vi "Dashboard Main.vi"() -> ()   [LabVIEW 2011]
uses:
  <vilib>/Rock Robotics/WPI/Camera/WPI_CameraImageSize.ctl
  Dashboard Datatype.ctl
  <vilib>/Rock Robotics/WPI/DriverStation/WPI_DriverStationDigitalData.ctl
  UDP Communication Folder/UDP Dashboard Packet TypeDef.ctl
panel:
  out "Turret Pot":dbl(knob) scale=0.0..5.0
  out "Right":bool
  out "Off":bool
  out "Left":bool
  in  "Tab Control":enum32{"Competition", "Debug"}(tab)
  out "Aligned":bool
  in  "RPM":dbl(slide)=-30.0 scale=-200.0..200.0 scale format="%#.2g"
  out "Warmup":bool
  out "Automatic Mode":bool
  out "Allow Fire":bool
  in  "Viewer":T1(tab)
  in  "Video Enable":bool=TRUE
  out "Camera Image":T2(plugin-control)
  out "Buttons 1":cluster{"1":bool, "2":bool, "3":bool}
  out "Kinect 1":cluster{"X":dbl, "Y":dbl, "Z":dbl} {"X" scale=1.0..-1.0; "Y" scale=1.0..-1.0; "Z" scale=1.0..-1.0}
  out "Buttons 2":cluster{"1":bool, "2":bool, "3":bool}
  out "Kinect 2":cluster{"X":dbl, "Y":dbl, "Z":dbl} {"X" scale=1.0..-1.0; "Y" scale=1.0..-1.0; "Z" scale=1.0..-1.0}
  out "Version":string
  out "Skeleton Picture":picture
  out "Players":i8
  out "Processed Image":T2(plugin-control)
  in  "Display Mask":bool
  in  "Particle Count Limit":i32=10
  in  "Image Size":T3=enum."320x240"
  out "Distance":dbl format="%.2g"
  out "Gear":i32 format="%#.0f"
  out "Camera Tracking":bool
  out "Gyro":dbl(knob) scale=0.0..360.0
  out "Gyro Angle":dbl
  out "# Balls":u32
  in  "?":T4(tab)
  out "Encoders":cluster{"Average":dbl, "Left":dbl, "Right":dbl}
  out "IR Values":T5
  out "UDP Reading":bool
  out "Turret Info":T6 {"Target Pot" scale=1.0..4.0; "Current Voltage" scale=1.0..4.0}
  out "Gyro Angle":dbl(knob) scale=0.0..360.0
  out "Shooter Info":T7
  out "Solenoids":T8
  out "Ball State Machine":T9
  in  "Display Mask":bool
  in  "Color Range":T10={"Hue"={"Lower"=120, "Upper"=137}, "Sat"={"Lower"=130, "Upper"=255}, " Luma"={"Lower"=100, "Upper"=255}}
  in  "Score Limits":T11={"Rect Coverage"=66.0, "Aspect Ratio"=70.0, "X Edge Strength"=40.0, "Y Edge Strength"=60.0}
  out "Camera Image 2":T2(plugin-control)
  out "Processed Image 2":T2(plugin-control)
  out "Tracking Setpoint":dbl
  in  "Tracking Constant":dbl=0.07
  in  "Tracking Tolerance":dbl=0.2
  in  "Color":u32(colorbox)=16711680
  in  "Left Offset Percentage":dbl=2.4
  out "Gyro Angle 2":dbl
  out "Tracking OUT":dbl
  out "Target Info":T12(array[cluster])
  out "Servo Positions In":cluster{"X":dbl, "Y":dbl}
  in  "Area Size Limit":i32=444
  in  "Decimation":i32=1
  in  "Shooter PID gains":T13={"proportional gain (Kc)"=0.0025, "integral time (Ti, min)"=0.007, "derivative time (Td, min)"=0.0}
  in  "Tracking PID gains":T13={"proportional gain (Kc)"=0.25, "integral time (Ti, min)"=0.01, "derivative time (Td, min)"=0.0015}
  in  "Shooter PID gains 2":T13={"proportional gain (Kc)"=0.0028, "integral time (Ti, min)"=0.0, "derivative time (Td, min)"=0.0}
  in  "Shooter Control":T14={"Manual Enabled"=FALSE, "Manual Distance"=0.0, "Power Constant"=0.0, "RPM Constant"=-30.0, "Layup Distance"=10.0, "RPM Range"={"Max Percentage"=1.005, "Min Percentage"=0.985}, "Dt In"=0.02}
  in  "Tracking Limit":dbl=0.55
  in  "Autonomous Ball Collection / Shoot Period":dbl=7.0
  out "8 -- Battery":sgl(graph)
  out "Analog Input":sgl[](array[slide]) scale=0.0..5.0
  out "Dashboard Datatype Warning":string="Warning: The Dashboard Datatype used by the robot project and this dashboard do not match.\nSee diagram for more details."
  out "Robot IP Address":string
  out "Image Error Message":string="Timeout in Camera Communications"
  out "Solenoid Output":bool[](array[boolean])
  out "PWM":cluster{u8, u8}[](array[slide])=[{0, 157}, {0, 157}, {0, 157}, {0, 157}, {0, 157}, {0, 157}, {0, 157}, {0, 157}, {0, 157}, {0, 169}] scale=1.0..255.0
  out "GPIO Output Enable":bool[](array[boolean])
  out "GPIO State":bool[](array[boolean])
  out "Relay":cluster{"Forward":bool[], "Reverse":bool[]}
  # "Layup"
  # "FAST - LONG"
  # "SLOW - SHORT"
  # "Gyro"
  # "SHOOTING PID"
  # "WARM UP PID"
  # "PID Values:\n   2.28.12:  0.003, 0, 0\n   3.2.12:    0.006, 0.000001, 0.0001\n   3.11.12:  0.0025, 0.009, 0\n   3.12.12: 0.0025, 0.007, 0"
  # "PID Values:\n   3.12.12: 2.5, 0.009, 0  Oscillating\n   3.12.12: 4.0, 0, 0         Steady state error\n\n   3.30.12: 0.03, 0.01, 0.002 (gyro)\n   4.26.12: 0.27, 0.01, 0.0018 (okay..)"
  # "PID Values:\n   3.12.12: 0.0028, 0, 0"
  # "Seconds"
  # "Limits tracking pid output"
  # "Analog #1"
  # "1"
  # "7"
  # "Communications"
  # "Solenoid #1"
  # "1"
  # "8"
  # "Digital #1"
  # "1"
  # "10"
  # "1"
  # "14"
  # "1"
  # "8"
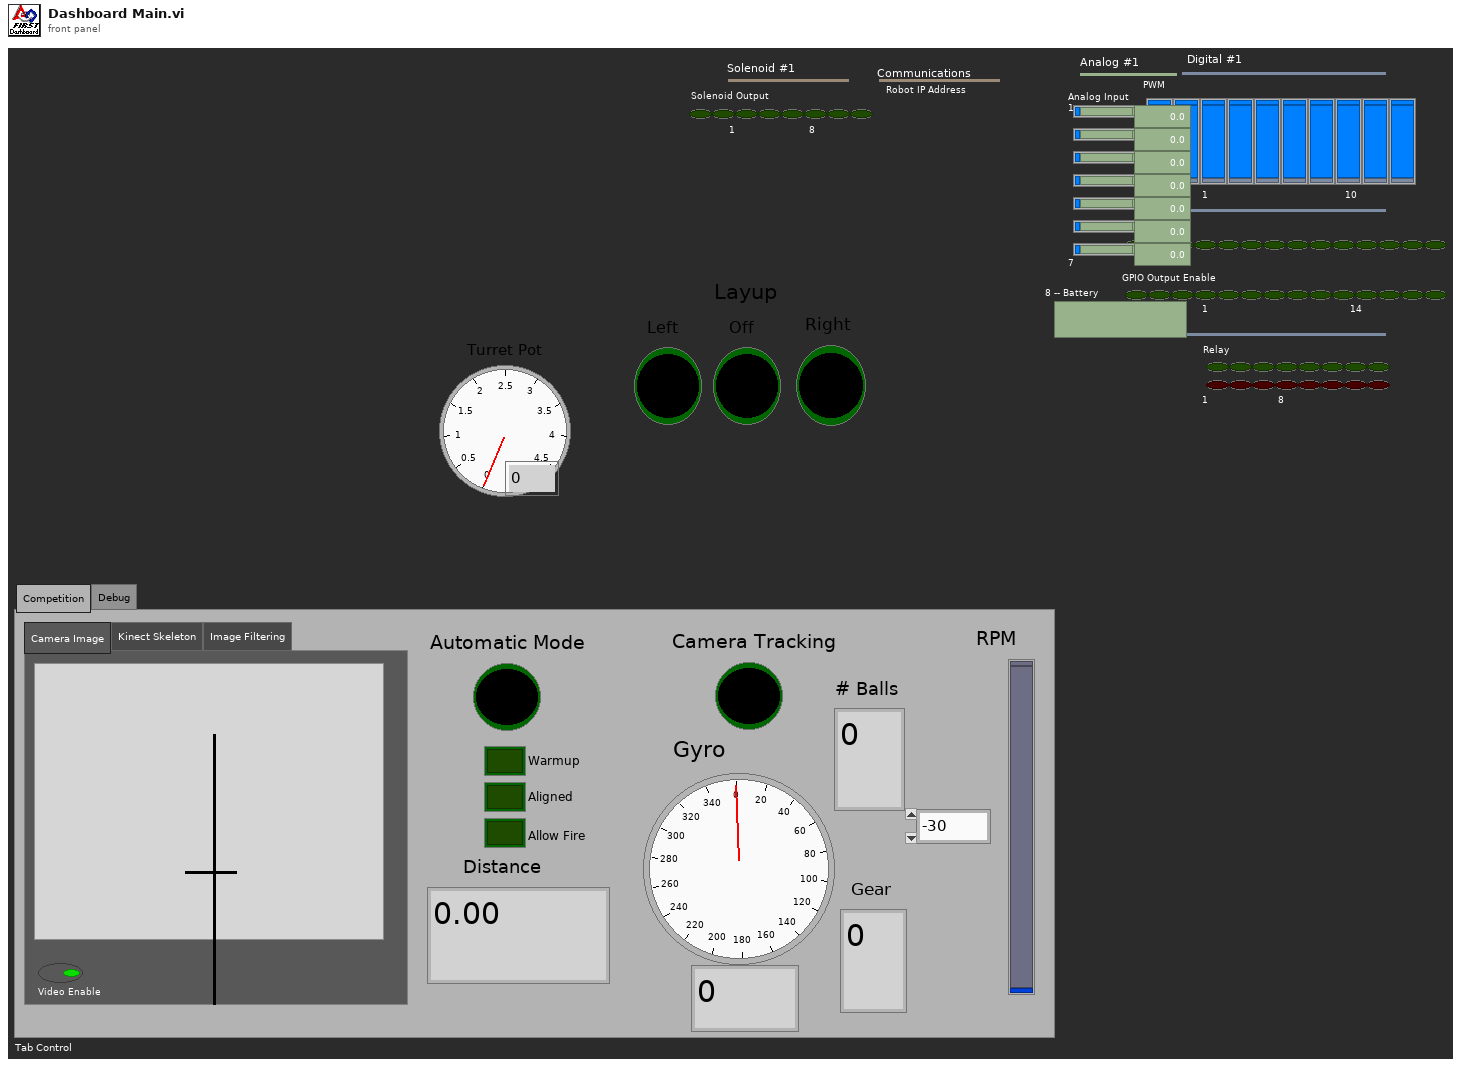
[diagram p1: front panel]
types:
  T1 = enum32{"Camera Image", "Kinect Skeleton", "Image Filtering"}
  T2 = typedef "IMAQ Image.ctl" = refnum<image>
  T3 = typedef "WPI_CameraImageSize.ctl" = enum16{"640x480", "320x240", "160x120"}
  T4 = enum32{"Sensors", "Vision Calib", "Vision Readings", "Numeric Controls"}
  T5 = cluster{"Front Roller":bool, "Back Roller":bool, "Lower Mag":bool, "Upper Mag":bool, "Front Enter":bool, "Rear Enter":bool}
  T6 = cluster{"Target Pot":dbl, "Motor Output":dbl, "Current Voltage":dbl}
  T7 = cluster{"Current RPM":dbl, "Distance Setpoint":dbl, "Target RPM":dbl, "Motor Output":dbl, "Base Power":dbl, "Dt Out":dbl}
  T8 = cluster{"Gear Shifter":bool, "Tipper":bool, "Tipper Lock":bool, "Stabilizer":bool}
  T9 = cluster{"Current State":u32, "Reading State":u32, "Number of Balls":u32, "State":enum16{"Load Balls", "Shoot", "Wait"}}
  T10 = cluster{"Hue":cluster{"Lower":i32, "Upper":i32}, "Sat":cluster{"Lower":i32, "Upper":i32}, " Luma":cluster{"Lower":i32, "Upper":i32}}
  T11 = cluster{"Rect Coverage":dbl, "Aspect Ratio":dbl, "X Edge Strength":dbl, "Y Edge Strength":dbl}
  T12 = cluster{"Position":cluster{"X":dbl, "Y":dbl}, "Distance (ft)":dbl}[]
  T13 = cluster{"proportional gain (Kc)":dbl, "integral time (Ti, min)":dbl, "derivative time (Td, min)":dbl}
  T14 = cluster{"Manual Enabled":bool, "Manual Distance":dbl, "Power Constant":dbl, "RPM Constant":dbl, "Layup Distance":dbl, "RPM Range":cluster{"Max Percentage":dbl, "Min Percentage":dbl}, "Dt In":dbl}
  T15 = typedef "UDP Dashboard Packet TypeDef.ctl" = cluster{"Distance":dbl, "Shooter Control":cluster{"Manual Enabled":bool, "Manual Distance":dbl, "Power Constant":dbl, "RPM Constant":dbl, "Layup Distance":dbl, "RPM Range":cluster{"Max Percentage":dbl, "Min Percentage":dbl}, "Dt In":dbl}, "Tracking Setpoint":dbl, "Shooter PID gains":cluster{"proportional gain (Kc)":dbl, "integral time (Ti, min)":dbl, "derivative time (Td, min)":dbl}, "Tracking PID gains":cluster{"proportional gain (Kc)":dbl, "integral time (Ti, min)":dbl, "derivative time (Td, min)":dbl}, "Shooter PID gains 2":cluster{"proportional gain (Kc)":dbl, "integral time (Ti, min)":dbl, "derivative time (Td, min)":dbl}, "Tracking Tolerance":dbl, "Tracking Limit":dbl, "Autonomous Ball Collection / Shoot Period":dbl}
  T16 = typedef "Dashboard Datatype.ctl" = cluster{cluster{"AnalogModule[0]":cluster{"Channel[0]":sgl, "Channel[1]":sgl, "Channel[2]":sgl, "Channel[3]":sgl, "Channel[4]":sgl, "Channel[5]":sgl, "Channel[6]":sgl, "Channel[7]":sgl}, "AnalogModule[1]":cluster{"Channel[0]":sgl, "Channel[1]":sgl, "Channel[2]":sgl, "Channel[3]":sgl, "Channel[4]":sgl, "Channel[5]":sgl, "Channel[6]":sgl, "Channel[7]":sgl}}, cluster{"DigitalModule[0]":T17, "DigitalModule[1]":T17}, "Solenoid":u8, "IR Values":cluster{"Front Roller":bool, "Back Roller":bool, "Lower Mag":bool, "Upper Mag":bool, "Front Enter":bool, "Rear Enter":bool}, "Solenoids":cluster{"Gear Shifter":bool, "Tipper":bool, "Tipper Lock":bool, "Stabilizer":bool}, "Allow Fire":bool, "Encoders":cluster{"Average":dbl, "Left":dbl, "Right":dbl}, "UDP Reading":bool, "Turret Info":cluster{"Target Pot":dbl, "Motor Output":dbl, "Current Voltage":dbl}, "Shooter Controls":cluster{"Shooter Warmup":bool, "Shooter Allow Fire":bool}, "Automatic Mode":bool, "Gyro Angle":dbl, "Servo Positions In":cluster{"X":dbl, "Y":dbl}, "Layup State":enum16{"Layup Left", "Layup Right", "Off"}, "Shooter Info":cluster{"Current RPM":dbl, "Distance Setpoint":dbl, "Target RPM":dbl, "Motor Output":dbl, "Base Power":dbl, "Dt Out":dbl}, "Tracking":bool, "Ball State Machine":cluster{"Current State":u32, "Reading State":u32, "Number of Balls":u32, "State":enum16{"Load Balls", "Shoot", "Wait"}}}
  T17 = typedef "WPI_DriverStationDigitalData.ctl" = cluster{"Relay Fwd":u8, "Relay Rev":u8, "GPIO":u16, "GPIO_OE":u16, "PWM":cluster{"PWM[0]":u8, "PWM[1]":u8, "PWM[2]":u8, "PWM[3]":u8, "PWM[4]":u8, "PWM[5]":u8, "PWM[6]":u8, "PWM[7]":u8, "PWM[8]":u8, "PWM[9]":u8}}
  T18 = typedef "Image Type" = u32
  T19 = cluster{"Competition mode":bool, "Robot Link":bool, "Autonomous":bool, "Enabled":bool, "E-Stop":bool}
  T20 = cluster{"AnalogModule[0]":cluster{"Channel[0]":sgl, "Channel[1]":sgl, "Channel[2]":sgl, "Channel[3]":sgl, "Channel[4]":sgl, "Channel[5]":sgl, "Channel[6]":sgl, "Channel[7]":sgl}, "AnalogModule[1]":cluster{"Channel[0]":sgl, "Channel[1]":sgl, "Channel[2]":sgl, "Channel[3]":sgl, "Channel[4]":sgl, "Channel[5]":sgl, "Channel[6]":sgl, "Channel[7]":sgl}}
  T21 = cluster{"DigitalModule[0]":T17, "DigitalModule[1]":T17}
  T22 = cluster{"Shooter Warmup":bool, "Shooter Allow Fire":bool}
  T23 = cluster{"Channel[0]":sgl, "Channel[1]":sgl, "Channel[2]":sgl, "Channel[3]":sgl, "Channel[4]":sgl, "Channel[5]":sgl, "Channel[6]":sgl, "Channel[7]":sgl}[]
  T24 = cluster{"Channel[0]":sgl, "Channel[1]":sgl, "Channel[2]":sgl, "Channel[3]":sgl, "Channel[4]":sgl, "Channel[5]":sgl, "Channel[6]":sgl, "Channel[7]":sgl}
  T25 = typedef "LVRectTypeDef.ctl" = cluster{"left":i16, "top":i16, "right":i16, "bottom":i16}
  T26 = typedef "SkeletonTrackState.ctl" = enum32{"NotTracked", "PositionOnly", "Tracked"}
  T27 = cluster{"TrackingState":u8[], "Position":cluster{"x":sgl, "y":sgl, "z":sgl}, cluster{"x":sgl, "y":sgl, "z":sgl, sgl}[], "TrackState":T26}
  T28 = cluster{cluster{"ScaledToPercentRange":dbl, "ScaledToPercentRange":dbl, "ScaledToPercentRange":dbl}, cluster{bool, bool, bool}}[]
  T29 = typedef "LVBoundsTypeDef.ctl" = cluster{"Width":u32, "Height":u32}
  T30 = cluster{cluster{"ScaledToPercentRange":dbl, "ScaledToPercentRange":dbl, "ScaledToPercentRange":dbl}, cluster{bool, bool, bool}}
  T31 = cluster{"ScaledToPercentRange":dbl, "ScaledToPercentRange":dbl, "ScaledToPercentRange":dbl}
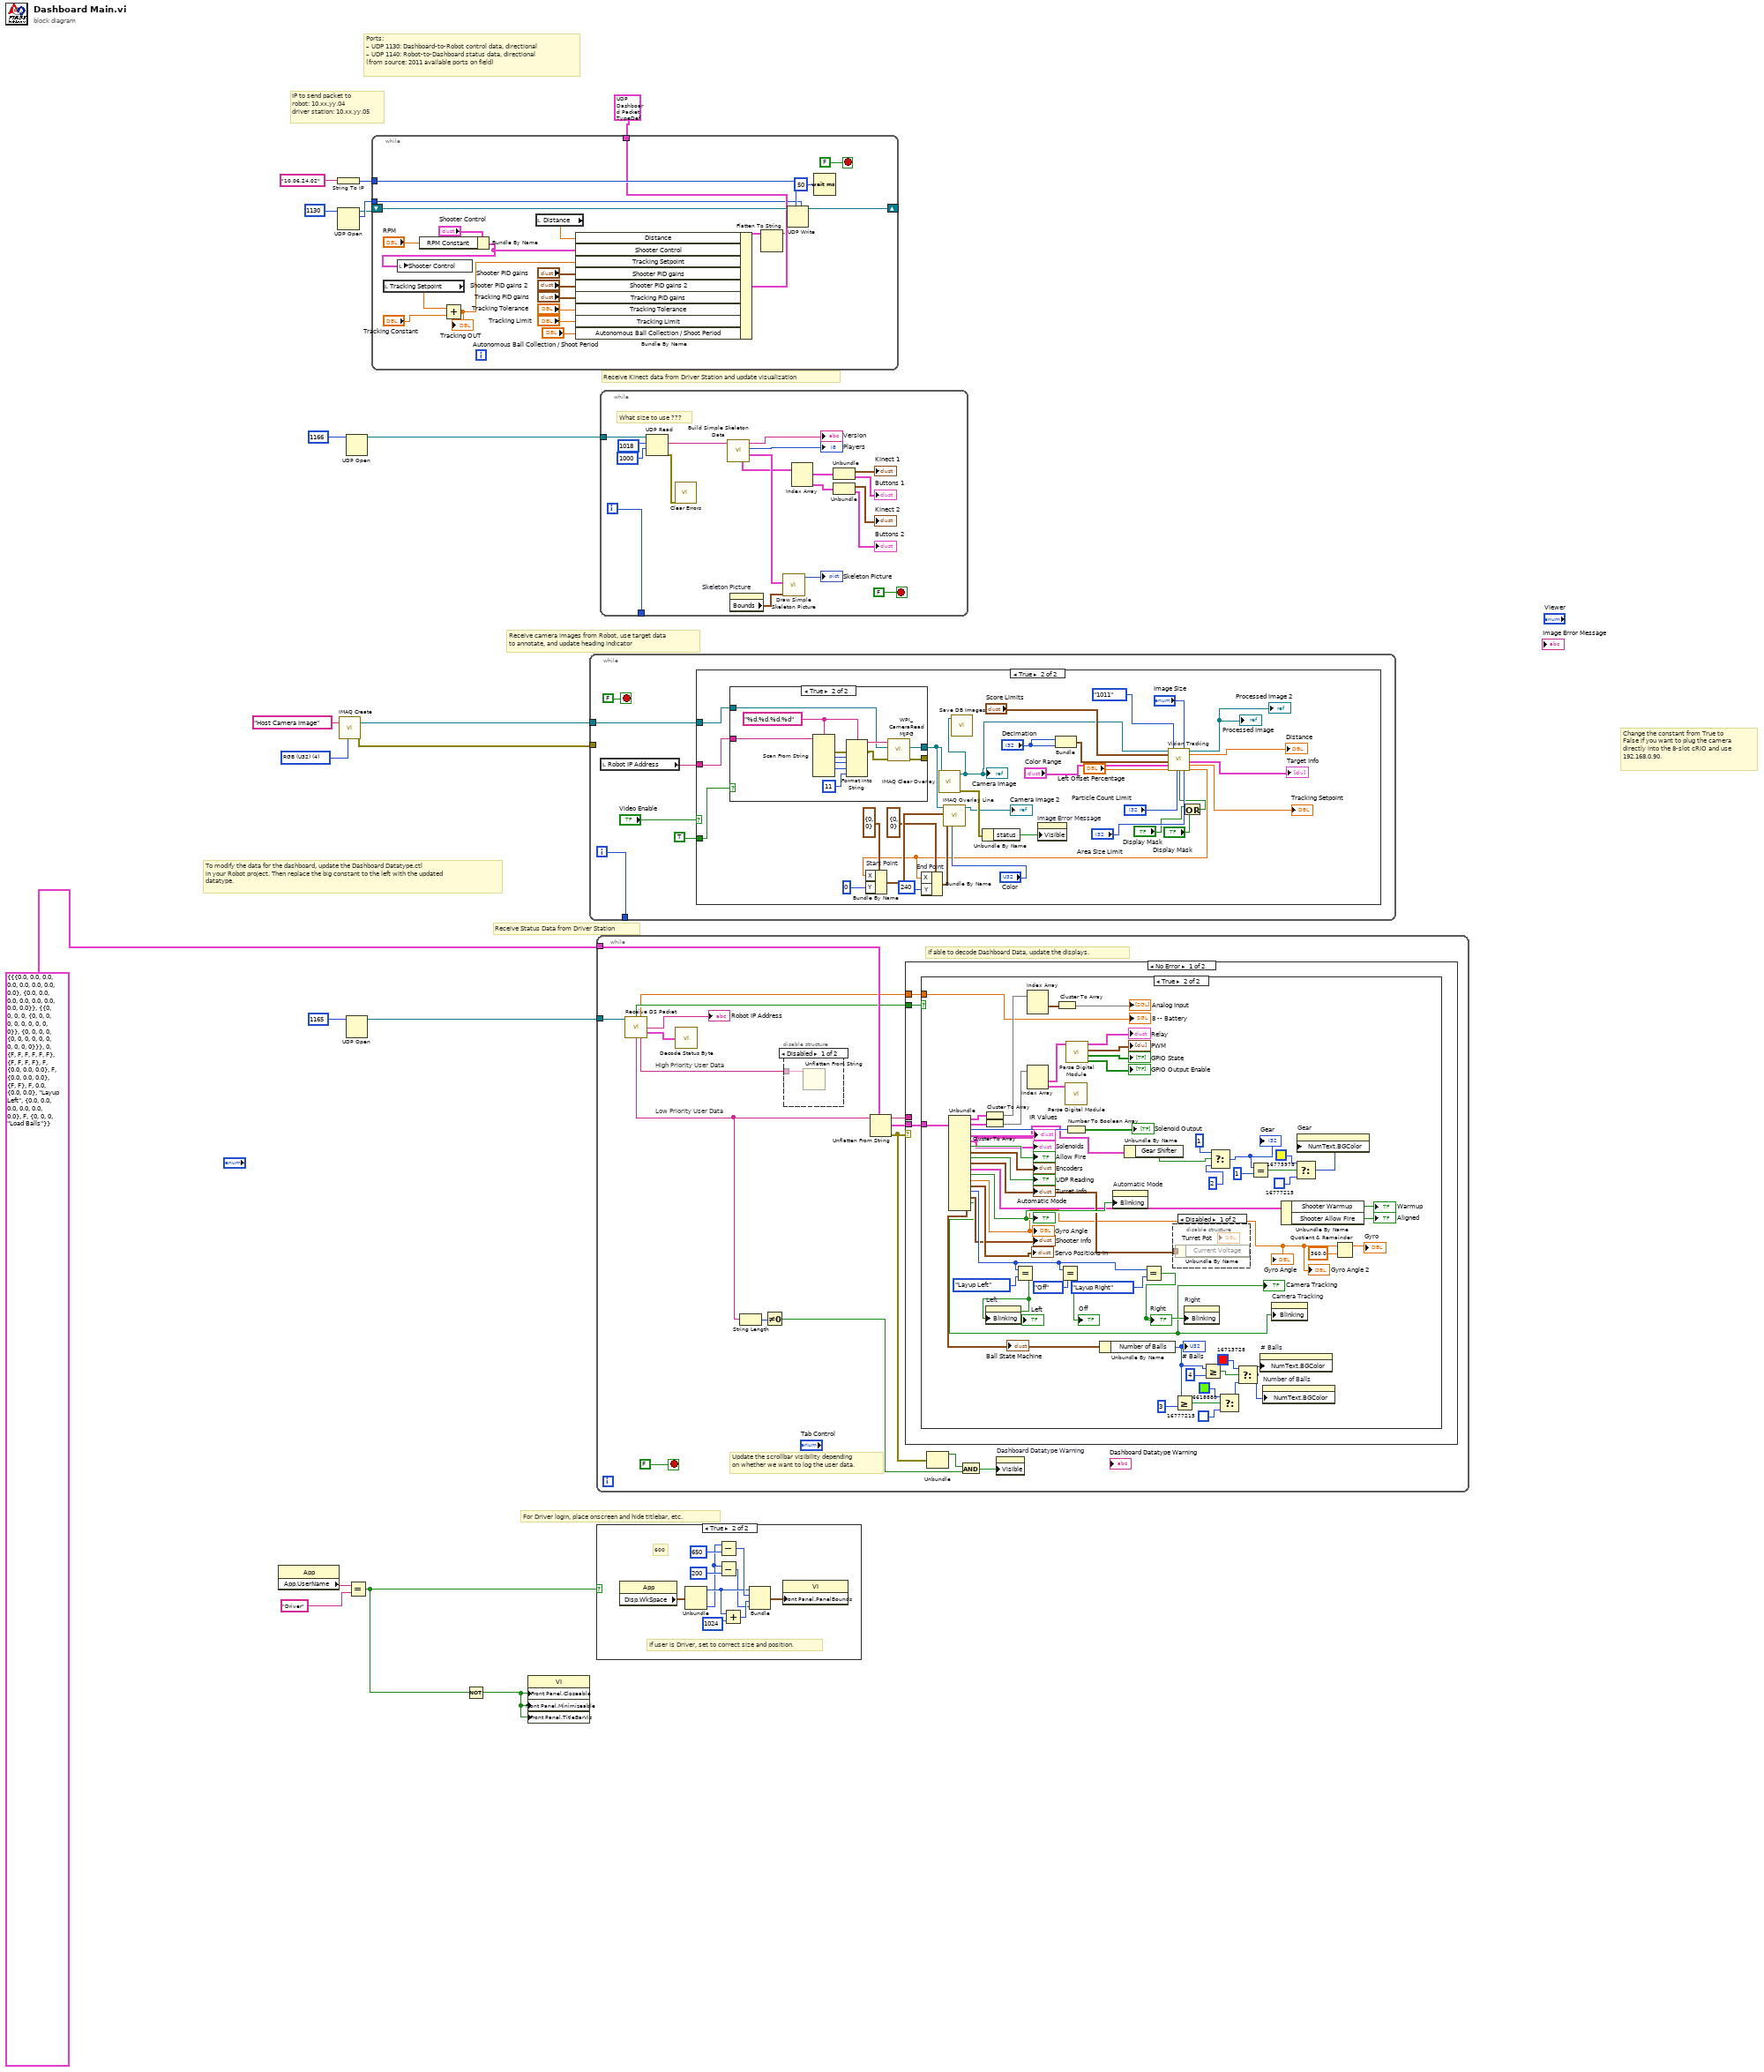
[diagram p0: block diagram]
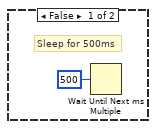
[diagram p7: hidden frame]
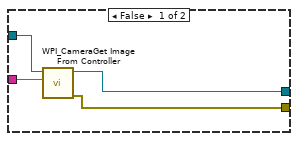
[diagram p8: hidden frame]
diagram:
  w17 = T18 4 items=["Grayscale (U8)", "Grayscale (I16)", "Grayscale (SGL)", "Complex (CSG)", "RGB (U32)", "HSL (U32)", "RGB (U64)"] ("Image Type")
  # "IP to send packet to \nrobot: 10.xx.yy.04\ndriver station: 10.xx.yy.05"
  # "Ports:\n– UDP 1130: Dashboard-to-Robot control data, directional\n– UDP 1140: Robot-to-Dashboard status data, directional\n(from source: 2011 available ports on field)"
  # "Change the constant from True to\nFalse if you want to plug the camera\ndirectly into the 8-slot cRIO and use\n192.168.0.90."
  # "Receive Kinect data from Driver Station and update visualization"
  # "For Driver login, place onscreen and hide titlebar, etc."
  # "To modify the data for the dashboard, update the Dashboard Datatype.ctl\nin your Robot project. Then replace the big constant to the left with the updated\ndatatype."
  # "Receive Status Data from Driver Station"
  # "Receive camera images from Robot, use target data\nto annotate, and update heading indicator"
  n1 = property class="App"() -> ("App.UserName"=w12:string)  [unwired: 2 in, 2 out]
  n2 = String To IP(1:"10.06.24.02") -> (0:w1:u32)
  n3 = UDP Open(11:u16 1130 ("port")) -> (port=w2:refnum<k16>, 2:w3:u16)  [unwired: 2 in, 3 out]
  n4 = call "IMAQ Create"("Image Name"="Host Camera Image", "Image Type"=w17) -> ("New Image"=w15:T2, "error out"=w14:errorcluster)  [unwired: 2 in, 1 out]
  n5 = UDP Open(11:u16 1166 ("port")) -> (port=w8:refnum<k16>)  [unwired: 2 in, 4 out]
  n6 = UDP Open(11:u16 1165 ("port")) -> (port=w18:refnum<k16>)  [unwired: 2 in, 4 out]
  n7 = Equal?(x=w12, y="Driver") -> (x = y?=w11:bool)
  n8 = while {
    tunnel: w1 -> [w39]
    tunnel: T15 {"Distance"=0.0, "Shooter Control"={"Manual Enabled"=FALSE, "Manual Distance"=0.0, "Power Constant"=0.0, "RPM Constant"=0.0, "Layup Distance"=0.0, "RPM Range"={"Max Percentage"=0.0, "Min Percentage"=0.0}, "Dt In"=0.0}, "Tracking Setpoint"=0.0, "Shooter PID gains"={"proportional gain (Kc)"=0.0, "integral time (Ti, min)"=0.0, "derivative time (Td, min)"=0.0}, "Tracking PID gains"={"proportional gain (Kc)"=0.0, "integral time (Ti, min)"=0.0, "derivative time (Td, min)"=0.0}, "Shooter PID gains 2"={"proportional gain (Kc)"=0.0, "integral time (Ti, min)"=0.0, "derivative time (Td, min)"=0.0}, "Tracking Tolerance"=0.0, "Tracking Limit"=0.0, "Autonomous Ball Collection / Shoot Period"=0.0} ("UDP Dashboard Packet") -> [w38]
    tunnel: w3 -> [w35]
    shift-right: [w34] -> _
    shift-left: w2 -> [w40]
    stop <- FALSE stop-if-true
    n9 = local read "Tracking Setpoint"() -> (w24:dbl)
    n10 = Bundle By Name(cluster="Shooter Control", "RPM Constant"="RPM") -> (w26:T14)
    n11 = local write "Shooter Control"(w26) -> ()
    n12 = Add(x=w24, y="Tracking Constant") -> (x+y=w23:dbl)
    "Tracking OUT" <- w23
    n13 = local read "Distance"() -> (w32:dbl)
    n14 = Bundle By Name(cluster=w38, "Distance"=w32, "Shooter Control"=w26, "Tracking Setpoint"=w23, "Shooter PID gains"="Shooter PID gains", "Shooter PID gains 2"="Shooter PID gains 2", "Tracking PID gains"="Tracking PID gains", "Tracking Tolerance"="Tracking Tolerance", "Tracking Limit"="Tracking Limit", "Autonomous Ball Collection / Shoot Period"="Autonomous Ball Collection / Shoot Period") -> (w37:T15)
    n15 = Flatten To String(anything=w37) -> (data string=w36:string)  [unwired: 3 in, 2 out]
    n16 = UDP Write(address=w39, port or service name=w35, connection ID=w40, data in=w36) -> (3:w34:refnum<k16>)  [unwired: 2 in, 1 out]
    n17 = Wait (ms)(milliseconds to wait=u32 50) -> ()  [unwired: 1 out]
  }
  n18 = Not(x=w11) -> (.not. x?=w10:bool)
  n19 = property class="VI"("Front Panel.Closeable"=w10, "Front Panel.Minimizeable"=w10, "Front Panel.TitleBarVis"=w10) -> ()  [unwired: 2 in, 2 out]
  n20 = while {
    tunnel: w15 -> [w45]
    tunnel: w14 -> [_]
    tunnel: [w42] -> _
    i -> [w42]
    stop <- FALSE stop-if-true
    n21 = local read "Robot IP Address"() -> (w46:string)
    n22 = case shown="True" "Video Enable" {
      tunnel: w46 -> [_ w80]
      tunnel: w45 -> [_ w79]
      tunnel: TRUE -> [_ w76]
      frame False {
        # "Sleep for 500ms"
        n23 = Wait Until Next ms Multiple(millisecond multiple=u32 500) -> ()  [unwired: 1 out]
      }
      frame True {
        n24 = case shown="True" w76 {
          tunnel: w79 -> [w83 w90]
          tunnel: [w81 w88] -> _
          tunnel: [w82 w89] -> w60
          tunnel: w80 -> [w84 w93]
          frame False {
            n25 = call <vilib>:"WPI_CameraGet Image From Controller.vi"("Controller Address"=w84, "Image"=w83) -> ("error out"=w81:errorcluster, "Image Out"=w82:T2)  [unwired: 2 in, 6 out]
          }
          frame True {
            w85 = "%d.%d.%d.%d" ("format string")
            n26 = Scan From String(format string=w85, input string=w93) -> (error out=w92:errorcluster, output 1=w94:i32, output 2=w95:i32, output 3=w96:i32)  [unwired: 2 in, 7 out]
            n27 = Format Into String(format string=w85, error in=w92, w94, w95, w96, 11 ("IP Suffix:")) -> (resulting string=w91:string, error out=w87:errorcluster)  [unwired: 1 in]
            n28 = call <vilib>:"WPI_CameraRead MJPG.vi"("error in"=w87, "Image"=w90, "address"=w91) -> ("error out"=w88:errorcluster, "Image Out"=w89:T2)  [unwired: 7 in]
          }
        }
        n29 = call "IMAQ Clear Overlay"("Image"=w60) -> ("error out"=w77:errorcluster, "Image Out"=w59:T2)  [unwired: 2 in, 7 out]
        "Camera Image" <- w59
        n30 = call "Save DB Images.vi"("Image"=w59) -> ()  [unwired: 2 in, 1 out]
        n31 = Unbundle By Name(w77) -> ("status"=w78:bool)
        n32 = property on="Image Error Message" class="Str"("Visible"=w78) -> ()  [unwired: 2 in, 2 out]
        n33 = Bundle("Decimation"="Decimation", "Decimation"="Decimation") -> (w69:cluster{"Decimation":i32, "Decimation":i32})  [unwired: 1 in]
        n34 = Or(x="Display Mask", y="Display Mask") -> (x .or. y?=w62:bool)
        n35 = call "Vision Tracking.vi"("Color Image In"=w59, "Score Limits"="Score Limits", "Decimate by"=w69, "Color Range"="Color Range", "Left Offset Percentage"="Left Offset Percentage", "Camera Type"=enum16{"206", "1011"}."1011", "Particle Count Limit"="Particle Count Limit", "Display Mask"=w62, "Image Size"="Image Size", "Area Size Limit"="Area Size Limit") -> ("Processed Image"=→"Processed Image" →"Processed Image 2":T2, "Distance (ft)"=→"Distance":dbl, "Target Info"=→"Target Info":T12, "Position.X"=→"Tracking Setpoint":dbl, "Center Line X"=w50:dbl)  [unwired: 5 in]
        n36 = Bundle By Name "Start Point"(cluster=cluster{"X":i32, "Y":i32} {"X"=0, "Y"=0} ("Start Point"), "X"=w50, "Y"=0) -> (w56:cluster{"X":i32, "Y":i32})
        n37 = Bundle By Name "End Point"(cluster=cluster{"X":i32, "Y":i32} {"X"=0, "Y"=0} ("End Point"), "X"=w50, "Y"=240) -> (w53:cluster{"X":i32, "Y":i32})
        n38 = call "IMAQ Overlay Line"("Color"="Color", "End Point"=w53, "Start Point"=w56, "Image"=w60) -> ("Image Out"=→"Camera Image 2":T2)  [unwired: 6 in, 1 out]
      }
    }
  }
  n39 = while {
    tunnel: w18 -> [w110]
    tunnel: T16 {{"AnalogModule[0]"={"Channel[0]"=0.0, "Channel[1]"=0.0, "Channel[2]"=0.0, "Channel[3]"=0.0, "Channel[4]"=0.0, "Channel[5]"=0.0, "Channel[6]"=0.0, "Channel[7]"=0.0}, "AnalogModule[1]"={"Channel[0]"=0.0, "Channel[1]"=0.0, "Channel[2]"=0.0, "Channel[3]"=0.0, "Channel[4]"=0.0, "Channel[5]"=0.0, "Channel[6]"=0.0, "Channel[7]"=0.0}}, {"DigitalModule[0]"={"Relay Fwd"=0, "Relay Rev"=0, "GPIO"=0, "GPIO_OE"=0, "PWM"={"PWM[0]"=0, "PWM[1]"=0, "PWM[2]"=0, "PWM[3]"=0, "PWM[4]"=0, "PWM[5]"=0, "PWM[6]"=0, "PWM[7]"=0, "PWM[8]"=0, "PWM[9]"=0}}, "DigitalModule[1]"={"Relay Fwd"=0, "Relay Rev"=0, "GPIO"=0, "GPIO_OE"=0, "PWM"={"PWM[0]"=0, "PWM[1]"=0, "PWM[2]"=0, "PWM[3]"=0, "PWM[4]"=0, "PWM[5]"=0, "PWM[6]"=0, "PWM[7]"=0, "PWM[8]"=0, "PWM[9]"=0}}}, "Solenoid"=0, "IR Values"={"Front Roller"=FALSE, "Back Roller"=FALSE, "Lower Mag"=FALSE, "Upper Mag"=FALSE, "Front Enter"=FALSE, "Rear Enter"=FALSE}, "Solenoids"={"Gear Shifter"=FALSE, "Tipper"=FALSE, "Tipper Lock"=FALSE, "Stabilizer"=FALSE}, "Allow Fire"=FALSE, "Encoders"={"Average"=0.0, "Left"=0.0, "Right"=0.0}, "UDP Reading"=FALSE, "Turret Info"={"Target Pot"=0.0, "Motor Output"=0.0, "Current Voltage"=0.0}, "Shooter Controls"={"Shooter Warmup"=FALSE, "Shooter Allow Fire"=FALSE}, "Automatic Mode"=FALSE, "Gyro Angle"=0.0, "Servo Positions In"={"X"=0.0, "Y"=0.0}, "Layup State"=enum."Layup Left", "Shooter Info"={"Current RPM"=0.0, "Distance Setpoint"=0.0, "Target RPM"=0.0, "Motor Output"=0.0, "Base Power"=0.0, "Dt Out"=0.0}, "Tracking"=FALSE, "Ball State Machine"={"Current State"=0, "Reading State"=0, "Number of Balls"=0, "State"=enum."Load Balls"}} ("Dashboard Data") -> [w109]
    stop <- FALSE stop-if-true
    # "High Priority User Data"
    # "Low Priority User Data"
    # "Update the scrollbar visibility depending\non whether we want to log the user data."
    # "If able to decode Dashboard Data, update the displays."
    n40 = call "Receive DS Packet.vi"("Recv Socket"=w110) -> ("New Dashboard Data"=w106:bool, "Battery"=w97:sgl, "Robot IP Address"=→"Robot IP Address":string, "Status"=w111:T19, "Low Priority User Data"=w99:string, "High Priority User Data"=w98:string)  [unwired: 1 in, 8 out]
    n41 = call "Decode Status Byte.vi"("Status Byte"=w111) -> ()  [unwired: 2 out]
    n42 = String Length(string=w99) -> (length=w101:i32)
    n43 = Not Equal To 0?(x=w101) -> (x != 0?=w104:bool)
    n44 = disable-structure shown="Disabled" {
      disable-tunnel: w98 -> [w113 _]
      frame Disabled {
        n45 = Unflatten From String(binary string=w113) -> ()  [unwired: 2 in, 5 out]
      }
      frame Enabled {
      }
    }
    n46 = Unflatten From String(type=w109, binary string=w99) -> (rest of the binary string=w102:string, value=w108:T16, error out=w107:errorcluster)  [unwired: 1 in, 2 out]
    n47 = case shown="No Error" w107 {
      tunnel: w108 -> [w116 _]
      tunnel: w106 -> [w115 _]
      tunnel: w102 -> [_ _]
      tunnel: w97 -> [w114 _]
      frame No Error {
        n48 = case shown="True" w115 {
          tunnel: w116 -> [_ w166]
          tunnel: w114 -> [_ w160]
          frame False {
            # "Don't update if the robot hasn't sent new data"
          }
          frame True {
            n49 = Unbundle(w166) -> (w163:T20, w164:T21, "Solenoid"=w165:u8, "IR Values"=→"IR Values":T5, "Solenoids"=w148:T8, "Allow Fire"=→"Allow Fire":bool, "Encoders"=→"Encoders":cluster{"Average":dbl, "Left":dbl, "Right":dbl}, "UDP Reading"=→"UDP Reading":bool, "Turret Info"=w141:T6, "Shooter Controls"=w140:T22, "Automatic Mode"=w142:bool, "Gyro Angle"=w134:dbl, "Servo Positions In"=→"Servo Positions In":cluster{"X":dbl, "Y":dbl}, "Layup State"=w151:enum16{"Layup Left", "Layup Right", "Off"}, "Shooter Info"=→"Shooter Info":T7, "Tracking"=w137:bool, "Ball State Machine"=w133:T9)
            "Turret Info" <- w141
            "Automatic Mode" <- w142
            "Gyro Angle" <- w134
            "Camera Tracking" <- w137
            "Solenoids" <- w148
            "Gyro Angle" <- w134
            "Gyro Angle 2" <- w134
            "Ball State Machine" <- w133
            n50 = Cluster To Array(cluster=w163) -> (array=w174:T23)
            n51 = Cluster To Array(cluster=w164) -> (array=w173:T17[])
            n52 = Equal?(x=w151, y=enum16{"Layup Left", "Layup Right", "Off"}."Layup Left" ("Layup State")) -> (x = y?=w143:bool)
            "Left" <- w143
            n53 = property on="Left" class="Bool (strict)"("Blinking"=w143) -> ()  [unwired: 2 in, 2 out]
            n54 = Index Array(array=w174) -> (element #1=w161:T24)  [unwired: 2 in, 1 out]
            n55 = Index Array(array=w173) -> (element #1=w172:T17, element #2=w167:T17)  [unwired: 2 in]
            n56 = Cluster To Array(cluster=w161) -> (array=→"Analog Input":sgl[])
            n57 = Equal?(x=w151, y=enum16{"Layup Left", "Layup Right", "Off"}."Off" ("Layup State")) -> (x = y?=→"Off":bool)
            n58 = call "Parse Digital Module.vi"("DigitalModule"=w167) -> ()  [unwired: 11 out]
            n59 = Number To Boolean Array(number=w165) -> (Boolean array=→"Solenoid Output":bool[])
            n60 = call "Parse Digital Module.vi"("DigitalModule"=w172) -> ("GPIO Output Enable"=→"GPIO Output Enable":bool[], "GPIO State"=→"GPIO State":bool[], "PWM"=→"PWM":cluster{u8, u8}[], "Relay"=→"Relay":cluster{"Forward":bool[], "Reverse":bool[]})  [unwired: 7 out]
            n61 = Unbundle By Name(w133) -> ("Number of Balls"=w126:u32)
            "# Balls" <- w126
            n62 = property on="Automatic Mode" class="Bool (strict)"("Blinking"=w142) -> ()  [unwired: 2 in, 2 out]
            n63 = Unbundle By Name(w148) -> ("Gear Shifter"=w145:bool)
            n64 = Equal?(x=w151, y=enum16{"Layup Left", "Layup Right", "Off"}."Layup Right" ("Layup State")) -> (x = y?=w144:bool)
            "Right" <- w144
            n65 = disable-structure shown="Disabled" {
              disable-tunnel: w141 -> [w176 _]
              frame Disabled {
                n66 = Unbundle By Name(w176) -> ("Current Voltage"=→"Turret Pot":dbl)
              }
              frame Enabled {
              }
            }
            n67 = Greater Or Equal?(x=w126, y=u32 3) -> (x >= y?=w130:bool)
            n68 = property on="Right" class="Bool (strict)"("Blinking"=w144) -> ()  [unwired: 2 in, 2 out]
            n69 = Greater Or Equal?(x=w126, y=u32 4) -> (x >= y?=w127:bool)
            n70 = Select(t=1, s=w145, f=2) -> (s? t:f=w118:i32)
            "Gear" <- w118
            n71 = Select(t=u32 6618880, s=w130, f=u32 16777215) -> (s? t:f=w128:u32)
            n72 = Select(t=u32 16713728, s=w127, f=w128) -> (s? t:f=w123:u32)
            n73 = Equal?(x=w118, y=1) -> (x = y?=w122:bool)
            n74 = property on="# Balls" class="DigNum (strict)"("NumText.BGColor"=w123) -> ()  [unwired: 2 in, 2 out]
            n75 = property on="Number of Balls" class="DigNum (strict)"("NumText.BGColor"=w123) -> ()  [unwired: 2 in, 2 out]
            n76 = property on="Camera Tracking" class="Bool (strict)"("Blinking"=w137) -> ()  [unwired: 2 in, 2 out]
            n77 = Unbundle By Name(w140) -> ("Shooter Warmup"=→"Warmup":bool, "Shooter Allow Fire"=→"Aligned":bool)
            n78 = Select(t=u32 16775978, s=w122, f=u32 16777215) -> (s? t:f=w117:u32)
            n79 = property on="Gear" class="DigNum (strict)"("NumText.BGColor"=w117) -> ()  [unwired: 2 in, 2 out]
            n80 = Quotient & Remainder(x=w134, y=360.0) -> (x-y*floor(x/y)=→"Gyro":dbl)  [unwired: 1 out]
            "8 -- Battery" <- w160
          }
        }
      }
      frame Error {
        # "Your datatypes don't match. The Dashboard Datatype.ctl in your Robot project\nand the big constant to the left of the loop need to match."
      }
    }
    n81 = Unbundle(w107) -> ("status"=w103:bool)  [unwired: 2 out]
    n82 = And(x=w103, y=w104) -> (x .and. y?=w105:bool)
    n83 = property on="Dashboard Datatype Warning" class="Str"("Visible"=w105) -> ()  [unwired: 2 in, 2 out]
  }
  n84 = case shown="True" w11 {
    frame False {
    }
    frame True {
      # "600"
      # "If user is Driver, set to correct size and position."
      n85 = property class="App"() -> ("Disp.WkSpace"=w187:T25)  [unwired: 2 in, 2 out]
      n86 = Unbundle(w187) -> ("left"=w182:i16, "bottom"=w178:i16)  [unwired: 2 out]
      n87 = Subtract(x=w178, y=650) -> (x-y=w184:i32)
      n88 = Subtract(x=w178, y=200) -> (x-y=w179:i32)
      n89 = Add(x=w182, y=1024) -> (x+y=w183:i32)
      n90 = Bundle("left"=w182, w184, w183, w179) -> (w186:cluster{"left":i16, i32, i32, i32})  [unwired: 1 out]
      n91 = property class="VI"("Front Panel.PanelBounds"=w186) -> ()  [unwired: 2 in, 2 out]
    }
  }
  n92 = while {
    tunnel: w8 -> [w204]
    tunnel: [w188] -> _
    i -> [w188]
    stop <- FALSE stop-if-true
    # "What size to use ???"
    n93 = UDP Read(connection ID=w204, max size (548)=1018 ("bytes to read"), timeout ms (25000)=1000) -> (data out=w198:string, error out=w196:errorcluster)  [unwired: 1 in, 3 out]
    n94 = call <vilib>:"Clear Errors.vi"("error in (no error)"=w196) -> ()  [unwired: 6 in, 1 out]
    n95 = call "Build Simple Skeleton Data.vi"("data out"=w198) -> ("Skeleton Data"=w199:T27, "NumPlayers"=→"Players":i8, "Version String"=→"Version":string, "Simple Joystick Info"=w195:T28)  [unwired: 6 in, 1 out]
    n96 = property on="Skeleton Picture" class="Pict"() -> ("Bounds"=w200:T29)  [unwired: 2 in, 2 out]
    n97 = call "Draw Simple Skeleton Picture.vi"("Bounds"=w200, "Simple Skeleton"=w199) -> ("new picture out"=→"Skeleton Picture":picture)  [unwired: 9 in]
    n98 = Index Array(array=w195) -> (element #1=w194:T30, element #2=w193:T30)  [unwired: 2 in]
    n99 = Unbundle(w194) -> (→"Kinect 1":T31, →"Buttons 1":cluster{bool, bool, bool})
    n100 = Unbundle(w193) -> (→"Kinect 2":T31, →"Buttons 2":cluster{bool, bool, bool})
  }
